vi "WebRequest.vi"(0 "API Key":string, 2 "JWT Token":string, 3 "client handle in":T1, 4 "URL":string, 5 "error in (no error)":errorcluster) -> (6 "body":string, 7 "error out":errorcluster, 8 "client handle out":T1)   [LabVIEW 2019]
uses:
  <vilib>/httpClient/ClientHandle.ctl
  <vilib>/httpClient/LabVIEWHTTPClient.lvlib
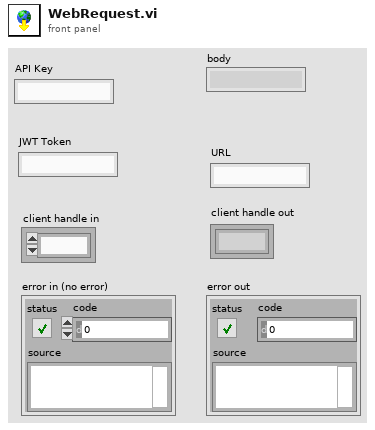
[diagram p1: front panel]
types:
  T1 = typedef "LabVIEWHTTPClient.lvlib/ClientHandle.ctl" = refnum<k1>
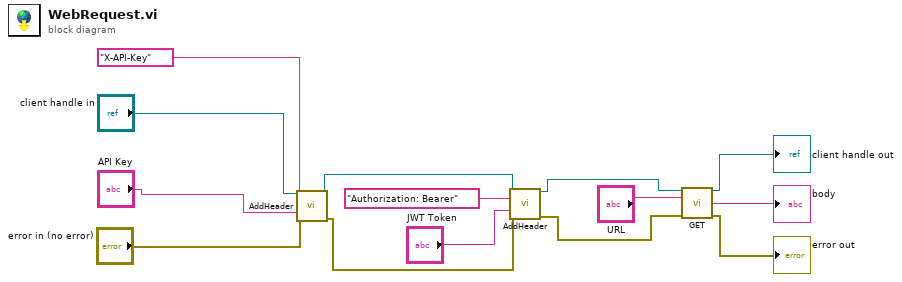
[diagram p0: block diagram]
diagram:
  n1 = call <vilib>:"AddHeader.vi"("client handle"="client handle in", "header"="X-API-Key", "value"="API Key", "error in (no error)"="error in (no error)") -> ("client handle out"=w9:T1, "error out"=w1:errorcluster)  [unwired: 10 in]
  n2 = call <vilib>:"AddHeader.vi"("client handle"=w9, "header"="Authorization: Bearer", "value"="JWT Token", "error in (no error)"=w1) -> ("client handle out"=w11:T1, "error out"=w12:errorcluster)  [unwired: 10 in]
  n3 = call <vilib>:"GET.vi"("client handle"=w11, "url"="URL", "error in (no error)"=w12) -> ("client handle out"=→"client handle out":T1, "body"=→"body":string, "error out"=→"error out":errorcluster)  [unwired: 9 in, 1 out]
